vi "Read Trace.vi"(7 "max points":i32, 8 "error in (no error)":errorcluster, 9 "time interval":T1, 10 "PG path":string, 11 "Data.PGQL in":refnum<class "Data.PGSQL.lvclass">) -> (0 "error out":errorcluster, 1 "Column (units)":string, 2 "Trace":cluster{timestamp[], dbl[]}, 3 "Data.PGSQL out":refnum<class "Data.PGSQL.lvclass">)   [LabVIEW 2013, in "Data.PGSQL.lvclass"]
uses:
  Data.PGSQL.lvclass
  Typedefs/Errors--enum.ctl
panel:
  out "resulting string":string
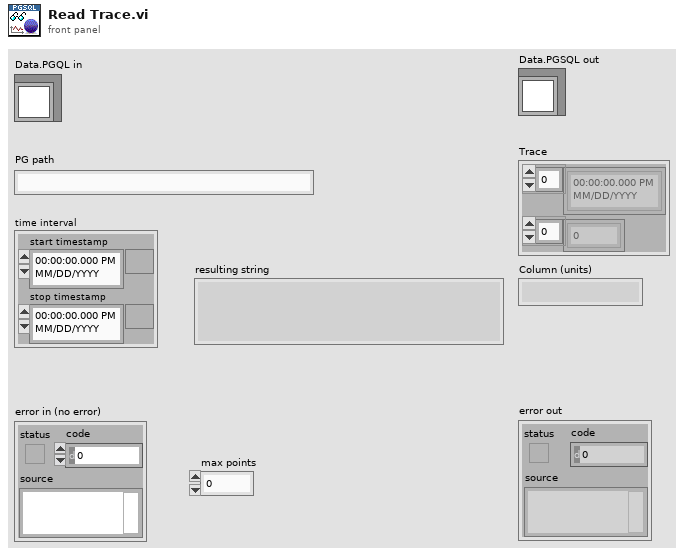
[diagram p1: front panel]
types:
  T1 = cluster{"start timestamp":timestamp, "stop timestamp":timestamp}
  T2 = typedef "Data.PGSQL.lvclass/Errors--enum.ctl" = enum16{"0: None", "5005: Path Type Not Supported", "5006: Number of Variables", "5008: Cannot write two data points", "5030: Start and End Times Identical", "5031: Input is not wholly", "5033: Bad path or paths", "5040: Invalid Instrument Name", "5050: Column can only hold string", "5051 Column can only hold bool", "5052: Column can only hold double", "5053: Column can only hold int"}
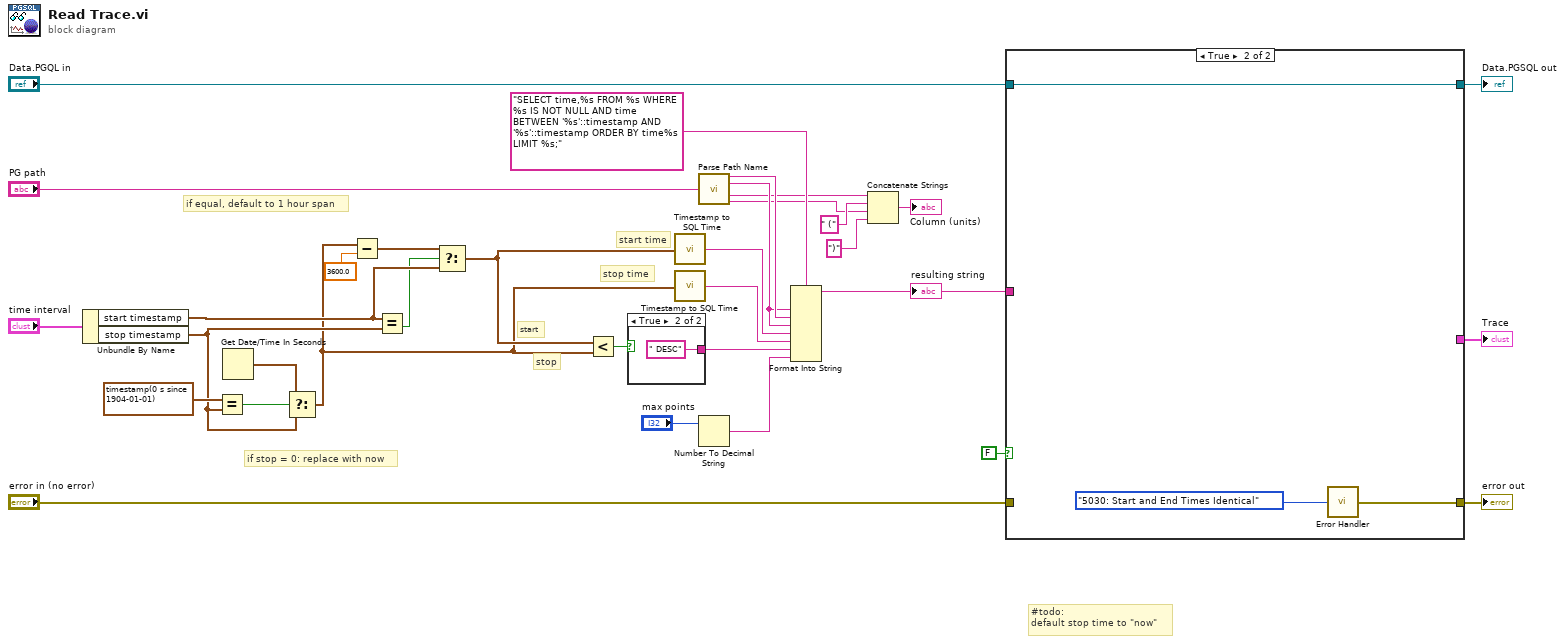
[diagram p0: block diagram]
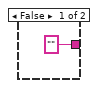
[diagram p2: hidden frame]
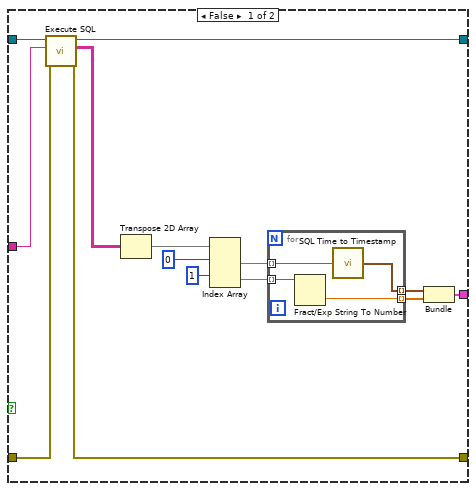
[diagram p3: hidden frame]
diagram:
  # "if equal, default to 1 hour span"
  # "if stop = 0: replace with now"
  # "stop"
  # "start"
  # "stop time"
  # "start time"
  # "#todo:\ndefault stop time to \"now\""
  n1 = Unbundle By Name("time interval") -> ("start timestamp"=w5:timestamp, "stop timestamp"=w6:timestamp)
  n2 = Equal?(x=timestamp(0 s since 1904-01-01) ("stop timestamp"), y=w6) -> (x = y?=w11:bool)
  n3 = Get Date/Time In Seconds() -> (seconds since 1Jan1904=w8:timestamp)
  n4 = Select(t=w8, s=w11, f=w6) -> (s? t:f=w1:timestamp)
  n5 = Subtract(x=w1, y=3600.0) -> (x-y=w7:timestamp)
  n6 = Equal?(x=w5, y=w6) -> (x = y?=w4:bool)
  n7 = Select(t=w7, s=w4, f=w5) -> (s? t:f=w2:timestamp)
  n8 = Less?(x=w2, y=w1) -> (x < y?=w33:bool)
  n9 = case shown="True" w33 {
    tunnel: ["" " DESC"] -> w28
    frame False {
    }
    frame True {
    }
  }
  n10 = call "Timestamp to SQL Time.vi"("seconds since 1Jan1904"=w2) -> ("date/time string"=w15:string)
  n11 = call "Timestamp to SQL Time.vi"("seconds since 1Jan1904"=w1) -> ("date/time string"=w14:string)
  n12 = call "Parse Path Name.vi"("PG Path"="PG path") -> ("Table path"=w24:string, "Column path"=w23:string, "Column name"=w21:string, "Column units"=w12:string)  [unwired: 10 in, 1 out]
  n13 = Number To Decimal String(number="max points") -> (decimal integer string=w29:string)  [unwired: 1 in]
  n14 = Format Into String(format string="SELECT time,%s FROM %s WHERE %s IS NOT NULL AND time BETWEEN '%s'::timestamp AND '%s'::timestamp ORDER BY time%s LIMIT %s;", w23, w24, w23, w15, w14, w28, w29) -> (resulting string=w19:string)  [unwired: 2 in, 1 out]
  "resulting string" <- w19
  n15 = Concatenate Strings(w21, " (" ("string"), w12, ")" ("string")) -> (→"Column (units)":string)
  n16 = case shown="True" FALSE {
    tunnel: [w42 _] -> w32
    tunnel: "Data.PGQL in" -> [w41 w56]
    tunnel: w19 -> [w37 _]
    tunnel: [w39 w54] -> w18
    tunnel: [w38 w56] -> w17
    tunnel: "error in (no error)" -> [w40 _]
    frame False {
      n17 = call "Execute SQL.vi"("error in"=w40, "SQL"=w37, "Data.PG"=w41) -> ("error out"=w39:errorcluster, "Result"=w36:string[][], "Data.PG out"=w38:refnum<class "Data.PGSQL.lvclass">)  [unwired: 6 in]
      n18 = Transpose 2D Array(2D array=w36) -> (transposed array=w49:string[][])
      n19 = Index Array(array=w49, index (row) #1=0 ("index (row)"), index (row) #2=1 ("index (row)")) -> (element #1=w46:string[], element #2=w45:string[])  [unwired: 2 in]
      n20 = for {
        tunnel: w46 -> [w53] mode=indexing
        tunnel: w45 -> [w52] mode=indexing
        tunnel: [w51] -> w43 mode=indexing
        tunnel: [w50] -> w44 mode=indexing
        n21 = Fract/Exp String To Number(string=w52) -> (number=w51:dbl)  [unwired: 3 in, 1 out]
        n22 = call "SQL Time to Timestamp.vi"("Get:Get String"=w53) -> ("Time Stamp"=w50:timestamp)
      }
      n23 = Bundle(w44, w43) -> (w42:cluster{timestamp[], dbl[]})  [unwired: 1 in]
    }
    frame True {
      n24 = call "Error Handler.vi"("Error code"=Errors--enum."5030: Start and End Times Identical") -> ("error out"=w54:errorcluster)
    }
  }
  "error out" <- w18
  "Trace" <- w32
  "Data.PGSQL out" <- w17
